vi "library path.vi"() -> (3 "Library Path":path=path "C:/Users/Daniel/Documents/nanomsg/lvnano/lvnanomsg.dll")   [LabVIEW 2013, in "lvnano.lvlib"]
uses:
  lvnano.lvlib
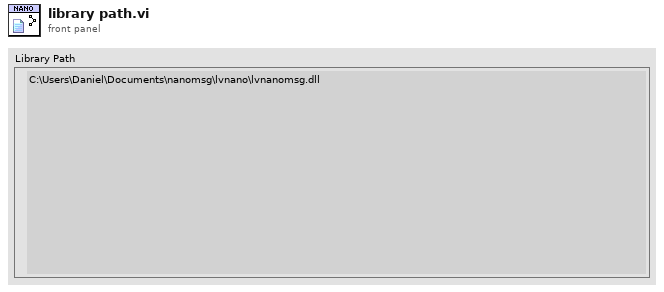
[diagram p1: front panel]
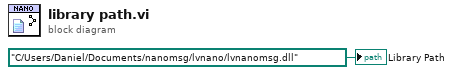
[diagram p0: block diagram]
diagram:
  "Library Path" <- path "C:/Users/Daniel/Documents/nanomsg/lvnano/lvnanomsg.dll" ("Library Path")
